vi "StellarNet Get-Set Channel Coefficients, ext precision.vi"(6 "Check sw.ini":bool, 7 "Number of Channels (from .dll)":i32=1, 8 "error in (no error)":errorcluster, 9 "Channel (1-based)":i32=1, 10 "Location of Spectrometer Coefficients xml file":path=path "C:/program files/StellarNet/SpectraWiz/StellarNet Spectrometer Coefficients.xml", 11 "Location of SpectraWiz ini file":path=path "C:/program files/StellarNet/SpectraWiz/sw.ini") -> (0 "error out":errorcluster, 3 "Coefficients":ext[](array[numeric]))   [LabVIEW 2023]
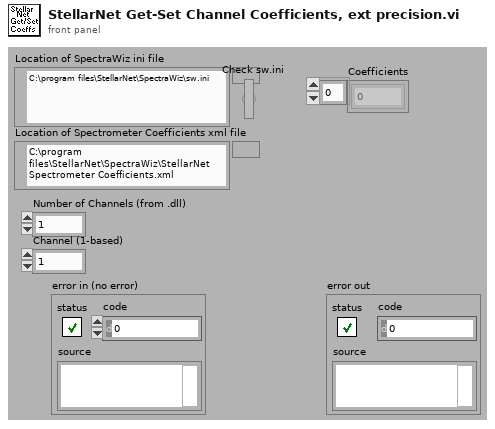
[diagram p1: front panel]
types:
  T1 = cluster{"Coefficients":ext[], "Wavelengths":dbl[]}[]
  T2 = cluster{"Coefficients":ext[], "Wavelengths":dbl[]}
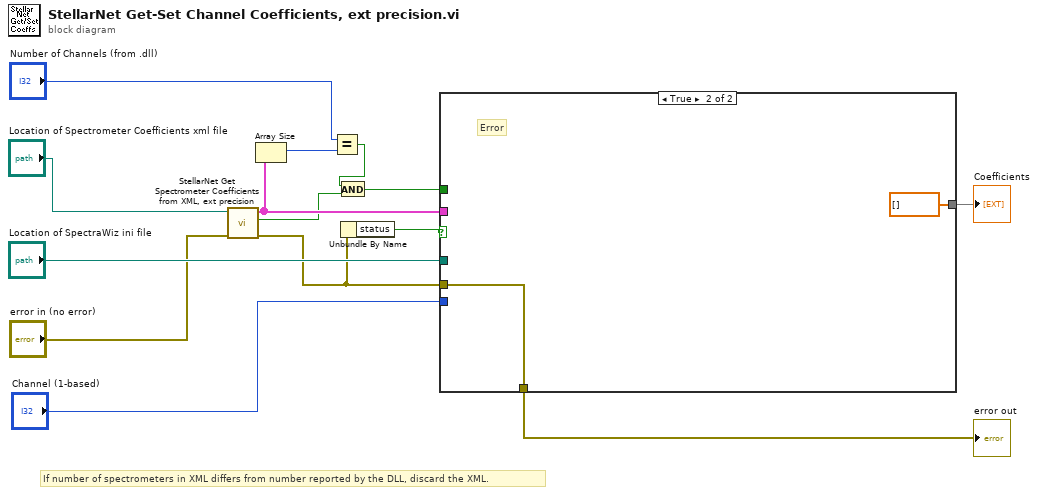
[diagram p0: block diagram]
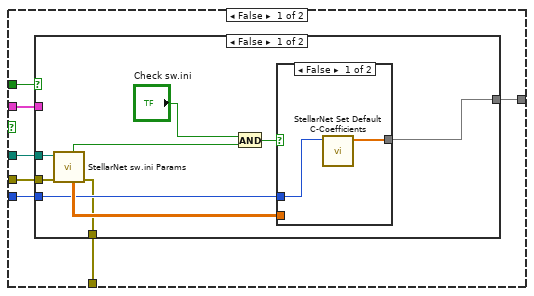
[diagram p2: hidden frame]
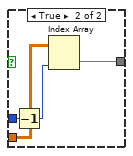
[diagram p3: hidden frame]
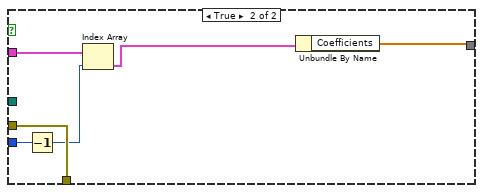
[diagram p4: hidden frame]
diagram:
  # "If number of spectrometers in XML differs from number reported by the DLL, discard the XML."
  n1 = call "StellarNet Get Spectrometer Coefficients from XML, ext precision.vi"("error in (no error)"="error in (no error)", "XML File Path"="Location of Spectrometer Coefficients xml file") -> ("error out"=w4:errorcluster, "file or folder exists?"=w12:bool, "Multi Channel Coeffs & WLs"=w14:T1)  [unwired: 7 in]
  n2 = Array Size(array=w14) -> (size(s)=w2:i32)
  n3 = Equal?(x="Number of Channels (from .dll)", y=w2) -> (x = y?=w13:bool)
  n4 = And(x=w13, y=w12) -> (x .and. y?=w11:bool)
  n5 = Unbundle By Name(w4) -> ("status"=w3:bool)
  n6 = case shown="True" w3 {
    tunnel: w4 -> [w21 w43]
    tunnel: w14 -> [w20 _]
    tunnel: w11 -> [w19 _]
    tunnel: "Location of SpectraWiz ini file" -> [w18 _]
    tunnel: "Channel (1-based)" -> [w17 _]
    tunnel: [w16 ext[] [] ("Coefficients")] -> w6
    tunnel: [w15 w43] -> w5
    frame False {
      n7 = case shown="False" w19 {
        tunnel: w21 -> [w30 w41]
        tunnel: w18 -> [w29 _]
        tunnel: w20 -> [_ w42]
        tunnel: w17 -> [w27 w38]
        tunnel: [w26 w39] -> w16
        tunnel: [w25 w41] -> w15
        frame False {
          n8 = call "StellarNet sw.ini Params.vi"("Error State (In)"=w30, "configuration file path"=w29) -> ("Error State (Out)"=w25:errorcluster, "Spectrometer Wavelengths"=w28:dbl[][], "file or folder exists?"=w23:bool)  [unwired: 3 in, 4 out]
          n9 = And(x="Check sw.ini", y=w23) -> (x .and. y?=w24:bool)
          n10 = case shown="False" w24 {
            tunnel: w28 -> [_ w36]
            tunnel: w27 -> [w31 w35]
            tunnel: [w32 w34] -> w26
            frame False {
              n11 = call "StellarNet Set Default C-Coefficients.vi"("Channel (1-based)"=w31) -> ("Coefficients"=w32:ext[])  [unwired: 10 in]
            }
            frame True {
              n12 = Decrement(x=w35) -> (x-1=w33:i32)
              n13 = Index Array(array=w36, index (col)=w33) -> (element=w34:dbl[])  [unwired: 1 in]
            }
          }
        }
        frame True {
          n14 = Decrement(x=w38) -> (x-1=w37:i32)
          n15 = Index Array(array=w42, index=w37) -> (element=w40:T2)
          n16 = Unbundle By Name(w40) -> ("Coefficients"=w39:ext[])
        }
      }
    }
    frame True {
      # "Error"
    }
  }
  "Coefficients" <- w6
  "error out" <- w5
